vi "Limit_FXP.vi"(7 "enabled":bool=TRUE, 8 "input valid":bool=TRUE, 10 "Limit":fxp<+/-,32,14>, 11 "Data in":fxp<+/-,32,14>[](array[numeric])=[0.0, 0.0]) -> (0 "output valid":bool, 3 "Data out":fxp<+/-,32,14>[](array[numeric]) format="%.23g")   [LabVIEW 2018]
uses:
  <vilib>/rvi/FXPMathLib/FxpDiv/subVIs/nifxpmath_Div_SimConfig.ctl
  <vilib>/rvi/FXPMathLib/FxpConvert/subVIs/nifxpmath_Convert_SimConfig.ctl
  <vilib>/fxp/LVFixedPointQuantizationPolicyTypeDef.ctl
  <vilib>/fxp/LVFixedPointOverflowPolicyTypeDef.ctl
  <vilib>/rvi/FXPMathLib/FxpSqrt/subVIs/nifxpmath_Sqrt_SimConfig.ctl
  <vilib>/rvi/FXPMathLib/FxpDiv/simVIs/DllFxpDivTemp_sub.vi
  <vilib>/rvi/FXPMathLib/FxpConvert/simVIs/DllFxpConvertTemp_sub.vi
  <vilib>/rvi/FXPMathLib/FxpSqrt/simVIs/DllSqrtTemp_sub.vi
  <vilib>/rvi/FXPMathLib/FxpDiv/XNode/nifxpmath_Div.xnode
  <vilib>/rvi/FXPMathLib/FxpConvert/XNode/nifxpmath_Convert.xnode
  <vilib>/rvi/FXPMathLib/FxpMul/XNode/nifxpmath_Multiplier.xnode
  <vilib>/rvi/FXPMathLib/FxpAdd/XNode/nifxpmath_Add.xnode
  <vilib>/rvi/FXPMathLib/FxpSqrt/XNode/nifxpmath_Sqrt.xnode
  <vilib>/rvi/FXPMathLib/sim/FxpSim.dll
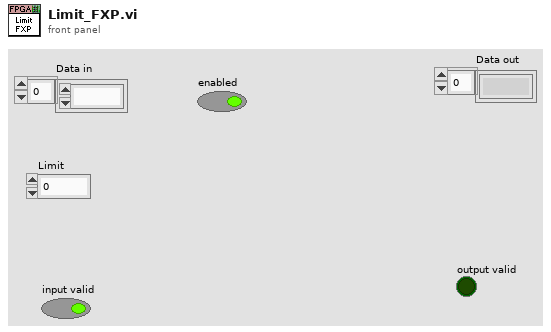
[diagram p1: front panel]
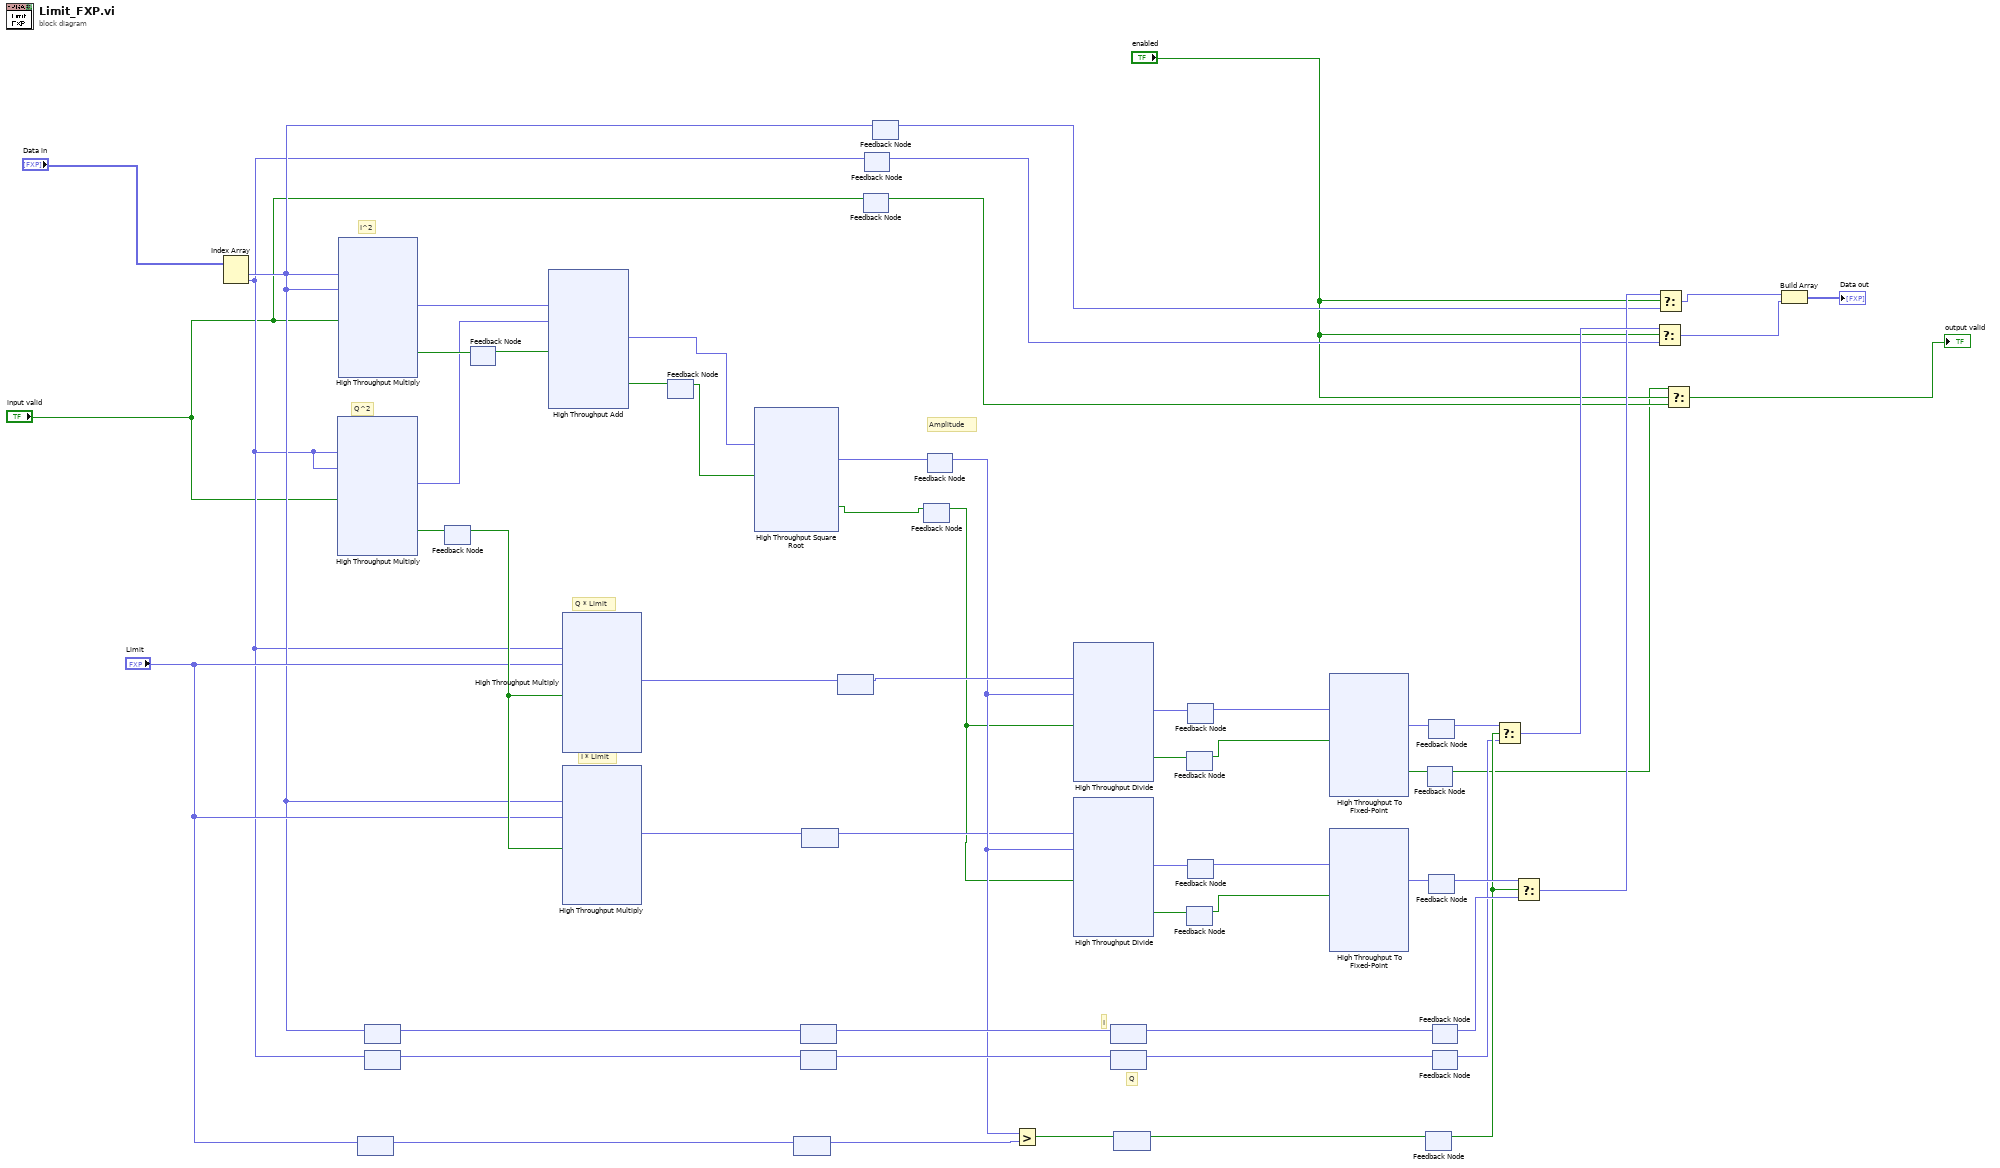
[diagram p0: block diagram]
diagram:
  # "Q"
  # "I"
  # "Q^2"
  # "I^2"
  # "I * Limit"
  # "Q * Limit"
  # "Amplitude"
  n1 = Index Array(array="Data in") -> (element #1=w13:fxp<+/-,32,14>, element #2=w12:fxp<+/-,32,14>)  [unwired: 2 in]
  n2 = xnode ("High Throughput Multiply")("x"=w12, "y"=w12, "input valid"="input valid") -> ("x*y"=w54:fxp<+/-,64,28>, "output valid"=w57:bool)  [unwired: 1 in, 1 out]
  n3 = xnode ("High Throughput Multiply")("x"=w13, "y"=w13, "input valid"="input valid") -> ("x*y"=w56:fxp<+/-,64,28>, "output valid"=w58:bool)  [unwired: 1 in, 1 out]
  n4 = feedback #1() -> (w35:fxp<+/-,32,14>)  [unwired: 1 in]
  n5 = feedback-in #1("Limit") -> ()
  n6 = feedback #2() -> (w37:fxp<+/-,32,14>)  [unwired: 1 in]
  n7 = feedback-in #2(w13) -> ()
  n8 = feedback #3() -> (w46:fxp<+/-,32,14>)  [unwired: 1 in]
  n9 = feedback-in #3(w12) -> ()
  n10 = feedback #4() -> (w39:bool)  [unwired: 1 in]
  n11 = feedback-in #4(w57) -> ()
  n12 = feedback #5() -> (w55:bool)  [unwired: 1 in]
  n13 = feedback-in #5(w58) -> ()
  n14 = xnode ("High Throughput Add")("x"=w56, "y"=w54, "input valid"=w55) -> ("x+y"=w50:fxp<+,64,28>, "output valid"=w53:bool)  [unwired: 1 in, 1 out]
  n15 = xnode ("High Throughput Multiply")("x"=w12, "y"="Limit", "input valid"=w39) -> ("x*y"=w49:fxp<+/-,64,28>)  [unwired: 1 in, 2 out]
  n16 = xnode ("High Throughput Multiply")("x"=w13, "y"="Limit", "input valid"=w39) -> ("x*y"=w32:fxp<+/-,64,28>)  [unwired: 1 in, 2 out]
  n17 = feedback #6() -> (w52:bool)  [unwired: 1 in]
  n18 = feedback-in #6(w53) -> ()
  n19 = xnode "High Throughput Square Root"("x"=w50, "input valid"=w52) -> ("sqrt(x)"=w47:fxp<+,64,14>, "output valid"=w51:bool)  [unwired: 1 in, 1 out]
  n20 = feedback #7() -> (w34:fxp<+/-,32,14>)  [unwired: 1 in]
  n21 = feedback-in #7(w35) -> ()
  n22 = feedback #8() -> (w38:fxp<+/-,32,14>)  [unwired: 1 in]
  n23 = feedback-in #8(w37) -> ()
  n24 = feedback #9() -> (w40:fxp<+/-,32,14>)  [unwired: 1 in]
  n25 = feedback-in #9(w46) -> ()
  n26 = feedback #10() -> (w27:fxp<+/-,64,28>)  [unwired: 1 in]
  n27 = feedback-in #10(w32) -> ()
  n28 = feedback #11() -> (w48:fxp<+/-,64,28>)  [unwired: 1 in]
  n29 = feedback-in #11(w49) -> ()
  n30 = feedback #12() -> (w4:bool)  [unwired: 1 in]
  n31 = feedback-in #12("input valid") -> ()
  n32 = feedback #13() -> (w6:fxp<+/-,32,14>)  [unwired: 1 in]
  n33 = feedback-in #13(w12) -> ()
  n34 = feedback #14() -> (w7:fxp<+/-,32,14>)  [unwired: 1 in]
  n35 = feedback-in #14(w13) -> ()
  n36 = feedback #15() -> (w26:bool)  [unwired: 1 in]
  n37 = feedback-in #15(w51) -> ()
  n38 = feedback #16() -> (w28:fxp<+,64,14>)  [unwired: 1 in]
  n39 = feedback-in #16(w47) -> ()
  n40 = Greater?(x=w28, y=w34) -> (0:w33:bool)
  n41 = xnode "High Throughput Divide"("x"=w48, "y"=w28, "input valid"=w26) -> ("x/y"=w43:fxp<+/-,64,14>, "output valid"=w45:bool)  [unwired: 1 in, 1 out]
  n42 = xnode "High Throughput Divide"("x"=w27, "y"=w28, "input valid"=w26) -> ("x/y"=w31:fxp<+/-,64,14>, "output valid"=w29:bool)  [unwired: 1 in, 1 out]
  n43 = feedback #17() -> (w22:fxp<+/-,32,14>)  [unwired: 1 in]
  n44 = feedback-in #17(w38) -> ()
  n45 = feedback #18() -> (w20:fxp<+/-,32,14>)  [unwired: 1 in]
  n46 = feedback-in #18(w40) -> ()
  n47 = feedback #19() -> (w23:bool)  [unwired: 1 in]
  n48 = feedback-in #19(w33) -> ()
  n49 = feedback #20() -> (w44:bool)  [unwired: 1 in]
  n50 = feedback-in #20(w45) -> ()
  n51 = feedback #21() -> (w30:bool)  [unwired: 1 in]
  n52 = feedback-in #21(w29) -> ()
  n53 = feedback #22() -> (w15:fxp<+/-,64,14>)  [unwired: 1 in]
  n54 = feedback-in #22(w43) -> ()
  n55 = feedback #23() -> (w14:fxp<+/-,64,14>)  [unwired: 1 in]
  n56 = feedback-in #23(w31) -> ()
  n57 = xnode "High Throughput To Fixed-Point"("x"=w15, "input valid"=w44) -> ("y"=w42:fxp<+/-,32,14>, "output valid"=w41:bool)  [unwired: 1 in, 1 out]
  n58 = xnode "High Throughput To Fixed-Point"("x"=w14, "input valid"=w30) -> ("y"=w25:fxp<+/-,32,14>)  [unwired: 1 in, 2 out]
  n59 = feedback #24() -> (w18:bool)  [unwired: 1 in]
  n60 = feedback-in #24(w23) -> ()
  n61 = feedback #25() -> (w2:bool)  [unwired: 1 in]
  n62 = feedback-in #25(w41) -> ()
  n63 = feedback #26() -> (w19:fxp<+/-,32,14>)  [unwired: 1 in]
  n64 = feedback-in #26(w42) -> ()
  n65 = feedback #27() -> (w24:fxp<+/-,32,14>)  [unwired: 1 in]
  n66 = feedback-in #27(w25) -> ()
  n67 = feedback #28() -> (w21:fxp<+/-,32,14>)  [unwired: 1 in]
  n68 = feedback-in #28(w22) -> ()
  n69 = feedback #29() -> (w17:fxp<+/-,32,14>)  [unwired: 1 in]
  n70 = feedback-in #29(w20) -> ()
  n71 = Select(t=w19, s=w18, f=w17) -> (s? t:f=w11:fxp<+/-,32,14>)
  n72 = Select(t=w24, s=w18, f=w21) -> (s? t:f=w9:fxp<+/-,32,14>)
  n73 = Select(t=w11, s="enabled", f=w6) -> (s? t:f=w10:fxp<+/-,32,14>)
  n74 = Select(t=w9, s="enabled", f=w7) -> (s? t:f=w8:fxp<+/-,32,14>)
  n75 = Select(t=w2, s="enabled", f=w4) -> (s? t:f=→"output valid":bool)
  n76 = Build Array(w8, w10) -> (→"Data out":fxp<+/-,32,14>[])
